vi "clear_log.vi"(8 "error in":errorcluster) -> (0 "error out":errorcluster)   [LabVIEW 2012]
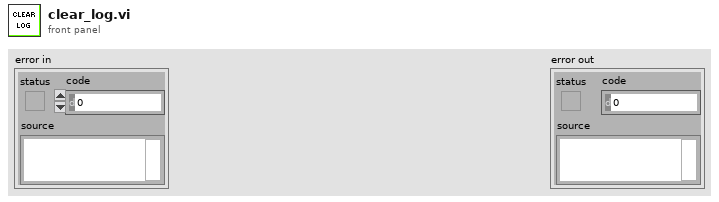
[diagram p1: front panel]
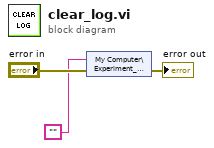
[diagram p0: block diagram]
diagram:
  n1 = shared-variable "My Computer\\Experiment_network_vars.lvlib\\Log"("", error in="error in") -> (error out=→"error out":errorcluster)
